vi "Aggregate Assertion Results.vi"(10 "Assertion Result":T1, 11 "Method Result In":T4) -> (3 "Method Result Out":T4)   [LabVIEW 2020, in "Method Result.lvlib"]
uses:
  Method Result.lvlib
  Assertion Result/Public/TypeDefs/Status.ctl
  Assertion Result/Assertion Result.lvlib
  Assertion Result/Public/TypeDefs/Assertion Type.ctl
  Assertion Result/Assertion Result.ctl
  Method Result.ctl
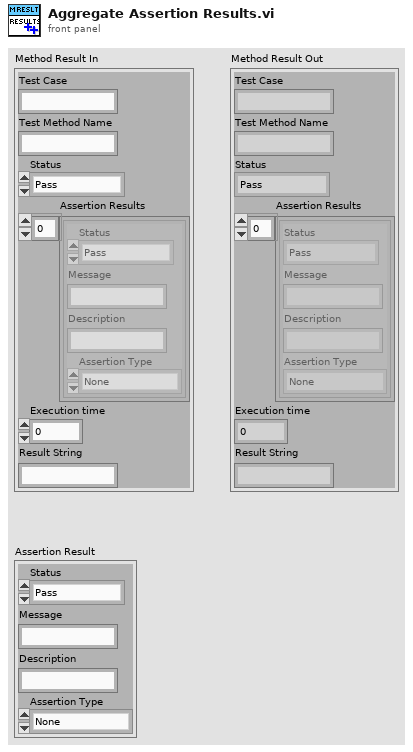
[diagram p1: front panel]
types:
  T1 = typedef "Assertion Result.lvlib/Assertion Result.ctl" = cluster{"Status":T2, "Message":string, "Description":string, "Assertion Type":T3}
  T2 = typedef "Assertion Result.lvlib/Status.ctl" = enum16{"Pass", "Fail", "Error", "Skipped", "Setup Error", "Broken", "Teardown Error"}
  T3 = typedef "Assertion Result.lvlib/Assertion Type.ctl" = enum16{"None", "Pass", "Fail", "Skip", "Pass if Equal", "Fail if Equal", "Pass if Error", "Fail if Error", "Pass if", "Fail if"}
  T4 = typedef "Method Result.lvlib/Method Result.ctl" = cluster{"Test Case":string, "Test Method Name":string, "Status":T2, "Assertion Results":T1[], "Execution time":dbl, "Result String":string}
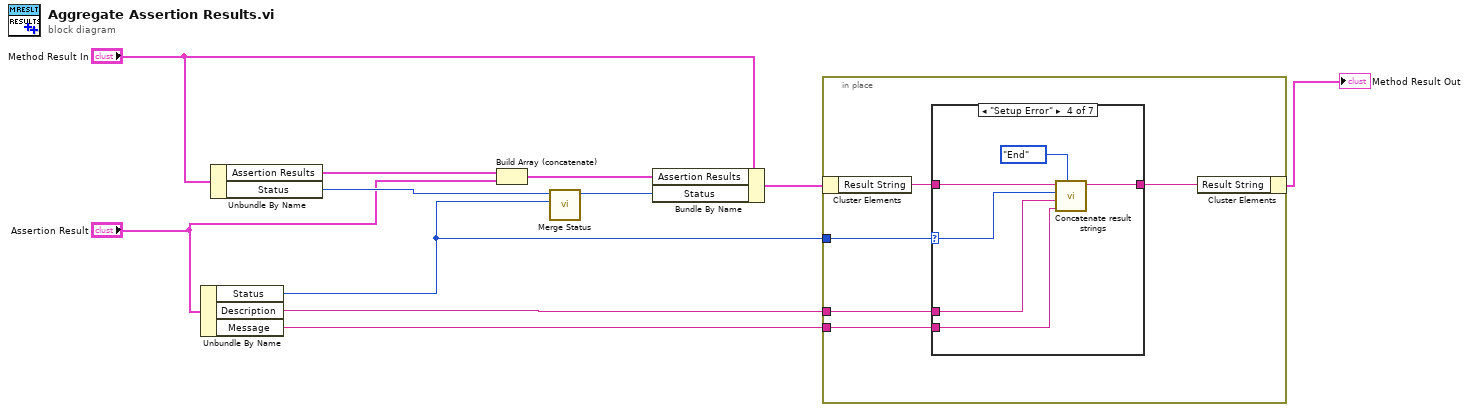
[diagram p0: block diagram]
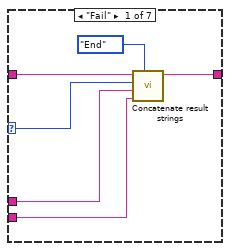
[diagram p2: hidden frame]
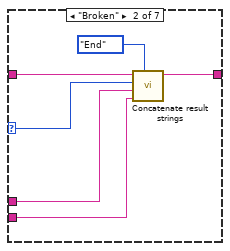
[diagram p3: hidden frame]
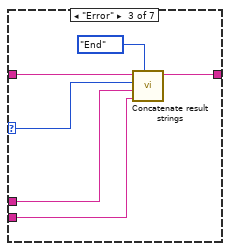
[diagram p4: hidden frame]
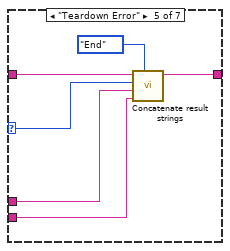
[diagram p5: hidden frame]
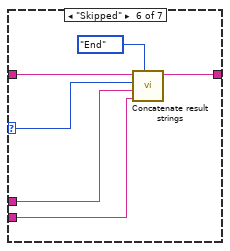
[diagram p6: hidden frame]
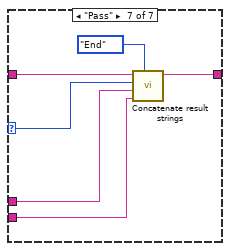
[diagram p7: hidden frame]
diagram:
  n1 = Unbundle By Name("Assertion Result") -> ("Status"=w2:T2, "Description"=w4:string, "Message"=w3:string)
  n2 = Unbundle By Name("Method Result In") -> ("Assertion Results"=w10:T1[], "Status"=w7:T2)
  n3 = Build Array (concatenate)(w10, "Assertion Result") -> (w9:T1[])
  n4 = call "Merge Status.vi"("New"=w2, "Current"=w7) -> ("Merged"=w6:T2)  [unwired: 8 in, 1 out]
  n5 = Bundle By Name(cluster="Method Result In", "Assertion Results"=w9, "Status"=w6) -> (w8:T4)
  n6 = in-place {
    in-place-border: w4 -> [w16]
    in-place-border: w2 -> [w13]
    in-place-border: w3 -> [w12]
    n7 = in-place-cluster #1(w8) -> ("Result String"=w15:string)
    n8 = case shown="\"Setup Error\"" w13 {
      selector: w13 -> [w19 w25 w31 w37 w43 w49 w55]
      tunnel: w16 -> [w22 w28 w34 w40 w46 w52 w58]
      tunnel: w15 -> [w21 w27 w33 w39 w45 w51 w57]
      tunnel: [w20 w26 w32 w38 w44 w50 w56] -> w14
      tunnel: w12 -> [w18 w24 w30 w36 w42 w48 w54]
      frame "Fail" {
        n9 = call "Concatenate result strings.vi"("Location"=enum16{"Start", "End"}."End", "Message"=w18, "Description"=w22, "Status"=w19, "Input String"=w21) -> ("Output String"=w20:string)  [unwired: 6 in]
      }
      frame "Broken" {
        n10 = call "Concatenate result strings.vi"("Location"=enum16{"Start", "End"}."End", "Message"=w24, "Description"=w28, "Status"=w25, "Input String"=w27) -> ("Output String"=w26:string)  [unwired: 6 in]
      }
      frame "Error" {
        n11 = call "Concatenate result strings.vi"("Location"=enum16{"Start", "End"}."End", "Message"=w30, "Description"=w34, "Status"=w31, "Input String"=w33) -> ("Output String"=w32:string)  [unwired: 6 in]
      }
      frame "Setup Error" {
        n12 = call "Concatenate result strings.vi"("Location"=enum16{"Start", "End"}."End", "Message"=w36, "Description"=w40, "Status"=w37, "Input String"=w39) -> ("Output String"=w38:string)  [unwired: 6 in]
      }
      frame "Teardown Error" {
        n13 = call "Concatenate result strings.vi"("Location"=enum16{"Start", "End"}."End", "Message"=w42, "Description"=w46, "Status"=w43, "Input String"=w45) -> ("Output String"=w44:string)  [unwired: 6 in]
      }
      frame "Skipped" {
        n14 = call "Concatenate result strings.vi"("Location"=enum16{"Start", "End"}."End", "Message"=w48, "Description"=w52, "Status"=w49, "Input String"=w51) -> ("Output String"=w50:string)  [unwired: 6 in]
      }
      frame "Pass" {
        n15 = call "Concatenate result strings.vi"("Location"=enum16{"Start", "End"}."End", "Message"=w54, "Description"=w58, "Status"=w55, "Input String"=w57) -> ("Output String"=w56:string)  [unwired: 6 in]
      }
    }
    n16 = in-place-cluster #1("Result String"=w14) -> (→"Method Result Out":T4)
  }
